vi "Predet_Sensor_Read_Setup(SubVI).vi"(8 "Error In":errorcluster, 9 "Temperature Freq":dbl, 10 "Sampling Time":dbl=1.0, 11 "Pressure Freq":dbl) -> (0 "error out":errorcluster, 1 "Pressure Samples":dbl, 2 "Temperature Samples":dbl, 3 "Temperature Task":refnum<k21>, 5 "Pressure Task":refnum<k21>)   [LabVIEW 2018]
uses:
  <vilib>/DAQmx/create/channels.llb/DAQmx Create Channel (AI-Current-Basic).vi
  <vilib>/DAQmx/create/channels.llb/DAQmx Create Channel (AI-Temperature-Thermocouple).vi
  <vilib>/DAQmx/configure/timing.llb/DAQmx Timing (Sample Clock).vi
  <resource>/objmgr/daqmx.rc
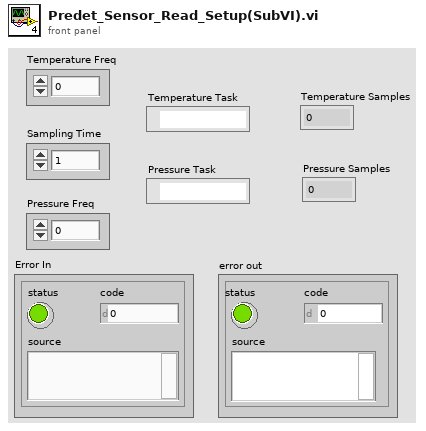
[diagram p1: front panel]
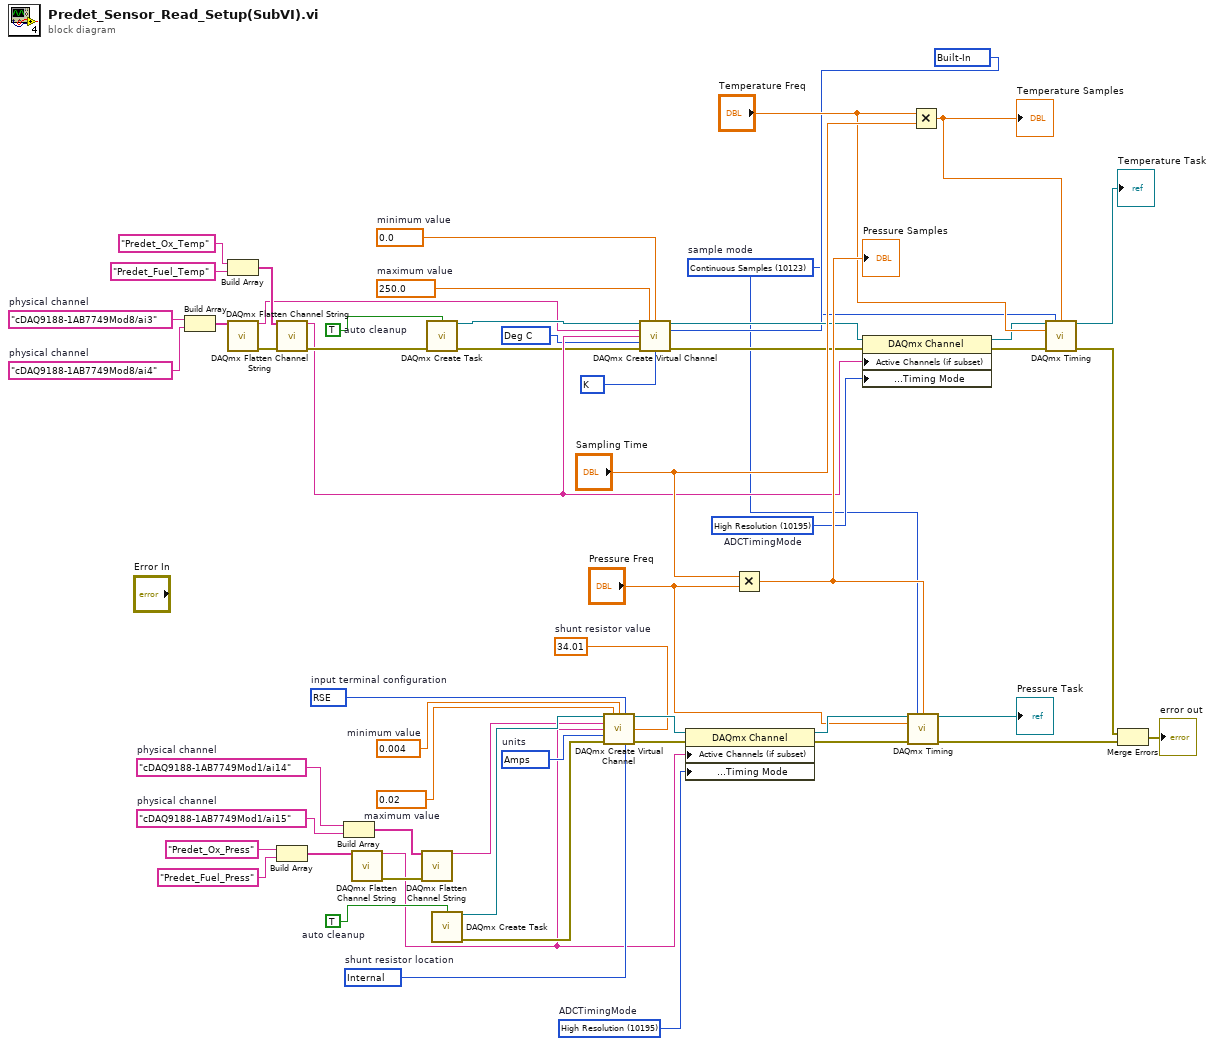
[diagram p0: block diagram]
diagram:
  w7 = "cDAQ9188-1AB7749Mod1/ai15"  # physical channel
  w8 = "cDAQ9188-1AB7749Mod1/ai14"  # physical channel
  w4 = 10123 items=["Finite Samples"=10178, "Continuous Samples"=10123, "Hardware Timed Single Point"=12522]  # sample mode
  w24 = 10195 items=["High Resolution"=10195, "High Speed"=14712, "Best 50 Hz Rejection"=14713, "Best 60 Hz Rejection"=14714]  # ADCTimingMode
  w23 = 10083 items=["default"=-1, "RSE"=10083, "NRSE"=10078, "Differential"=10106, "Pseudodifferential"=12529]  # input terminal configuration
  w22 = 10342 items=["Amps"=10342, "From Custom Scale"=10065]  # units
  w21 = 34.01  # shunt resistor value
  w20 = 10200 items=["Internal"=10200, "External"=10167]  # shunt resistor location
  w18 = 0.004  # minimum value
  w17 = 0.02  # maximum value
  w15 = TRUE  # auto cleanup
  w28 = "cDAQ9188-1AB7749Mod8/ai4"  # physical channel
  w29 = "cDAQ9188-1AB7749Mod8/ai3"  # physical channel
  w30 = 10143 items=["Deg C"=10143, "Deg F"=10144, "Kelvins"=10325, "Deg R"=10145, "From Custom Scale"=10065] ("units")
  w31 = 10073 items=["J"=10072, "K"=10073, "N"=10077, "R"=10082, "S"=10085, "T"=10086, "B"=10047, "E"=10055] ("thermocouple type")
  w32 = 10200 items=["Built-In"=10200, "Constant Value"=10116, "Channel"=10113] ("cjc source")
  w41 = 10195 items=["High Resolution"=10195, "High Speed"=14712, "Best 50 Hz Rejection"=14713, "Best 60 Hz Rejection"=14714]  # ADCTimingMode
  w38 = 0.0  # minimum value
  w37 = 250.0  # maximum value
  w35 = TRUE  # auto cleanup
  n1 = Build Array(w29, w28) -> (w27:string[])
  n2 = Build Array("Predet_Ox_Temp" ("name to assign"), "Predet_Fuel_Temp" ("name to assign")) -> (w46:string[])
  n3 = call <vilib>:"DAQmx Flatten Channel String.vi"("names in"=w27) -> ("names out"=w33:string, "error out"=w55:errorcluster)  [unwired: 13 in]
  n4 = call <vilib>:"DAQmx Flatten Channel String.vi"("names in"=w46, "error in"=w55) -> ("names out"=w47:string, "error out"=w48:errorcluster)  [unwired: 12 in]
  n5 = Build Array("Predet_Ox_Press" ("name to assign"), "Predet_Fuel_Press" ("name to assign")) -> (w12:string[])
  n6 = Build Array(w8, w7) -> (w6:string[])
  n7 = call <vilib>:"DAQmx Flatten Channel String.vi"("names in"=w12) -> ("names out"=w11:string, "error out"=w54:errorcluster)  [unwired: 13 in]
  n8 = call <vilib>:"DAQmx Flatten Channel String.vi"("names in"=w6, "error in"=w54) -> ("names out"=w13:string)  [unwired: 12 in, 1 out]
  n9 = call <vilib>:"DAQmx Create Task.vi"("auto cleanup"=w35, "error in"=w48) -> ("task out"=w36:refnum<k21>, "error out"=w34:errorcluster)  [unwired: 3 in, 9 out]
  n10 = call <vilib>:"DAQmx Create Task.vi"("auto cleanup"=w15) -> ("task out"=w16:refnum<k21>, "error out"=w14:errorcluster)  [unwired: 4 in, 9 out]
  n11 = call-poly <vilib>:"DAQmx Create Virtual Channel.vi"("task in"=w16, "maximum value"=w17, "minimum value"=w18, "input terminal configuration"=w23, "physical channels"=w13, "name to assign"=w11, "external shunt resistor value"=w21, "units"=w22, "error in"=w14, "shunt resistor location"=w20) -> ("task out"=w25:refnum<k21>, "error out"=w19:errorcluster)  [unwired: 1 in, 3 out]
  n12 = call-poly <vilib>:"DAQmx Create Virtual Channel.vi"("task in"=w36, "maximum value"=w37, "minimum value"=w38, "physical channels"=w33, "cjc source"=w32, "name to assign"=w47, "units"=w30, "error in"=w34, "thermocouple type"=w31) -> ("task out"=w42:refnum<k21>, "error out"=w39:errorcluster)  [unwired: 5 in]
  n13 = property class="DAQmx Channel"(reference=w25, error in=w19, "Active Channels (if subset)"=w11, "Analog Input:General Properties:Digitizer/ADC:Timing Mode"=w24) -> (reference out=w56:refnum<k21>, error out=w57:errorcluster)
  n14 = Multiply(x="Sampling Time", y="Pressure Freq") -> (x*y=w52:dbl)
  "Pressure Samples" <- w52
  n15 = property class="DAQmx Channel"(reference=w42, error in=w39, "Active Channels (if subset)"=w47, "Analog Input:General Properties:Digitizer/ADC:Timing Mode"=w41) -> (reference out=w43:refnum<k21>, error out=w40:errorcluster)
  n16 = call-poly <vilib>:"DAQmx Timing.vi"("task/channels in"=w56, "sample mode"=w4, "samples per channel"=w52, "rate"="Pressure Freq", "error in"=w57) -> ("task out"=→"Pressure Task":refnum<k21>, "error out"=w2:errorcluster)  [unwired: 2 in, 7 out]
  n17 = Multiply(x="Temperature Freq", y="Sampling Time") -> (x*y=w51:dbl)
  "Temperature Samples" <- w51
  n18 = call-poly <vilib>:"DAQmx Timing.vi"("task/channels in"=w43, "sample mode"=w4, "samples per channel"=w51, "rate"="Temperature Freq", "error in"=w40) -> ("task out"=→"Temperature Task":refnum<k21>, "error out"=w1:errorcluster)  [unwired: 2 in, 7 out]
  n19 = Merge Errors(w1, w2) -> (→"error out":errorcluster)
